vi "GUI_DG535_v2.0.0.vi"() -> ()   [LabVIEW 2020]
uses:
  Device Drivers/DG535/SubVis/mode_typDef.ctl
  Device Drivers/DG535/SubVis/load_typdef.ctl
  DelayControl_For Multiple Channels_535.ctl
  Device Drivers/DG535/SubVis/channels_TypDef_DG535.ctl
  GUI_DG645/DelayControl2.ctl
  Device Drivers/DG645/subVIs/polarity_TypDEf.ctl
  Shared/GUI_Template/GUI_master/tcp_new_data_event.ctl
  Shared/GUI_Template/GUI_master/tcp new data cluster.ctl
panel:
  out "tcp data event":T1
  in  "GUIdevice 1":string="P2-AndorCam"
  in  "stop":bool
  out "UDP error message":string caption="Device Errors"
  in  "Tab Control":T2(tab)
  in  "mode.Channel_C::1":T3
  in  "load.Channel_C::1":T4=enum."50 Ohm" caption="Impedance"
  in  "Delay.Channel_C":T5={"Channel"="C", "reference"=enum."T0", "delay"=0.01} {"delay" format="%+.12f"}
  in  "amplitude.Channel_C::1":dbl=4.0 caption="Amplitude (V)" min=-3.0 max=4.0
  in  "polarity.Channel_C::1":T8=enum."Positive" caption="Polarity"
  in  "mode.Channel_A::1":T3
  in  "load.Channel_A::1":T4=enum."50 Ohm" caption="Impedance"
  in  "Delay.Channel_A":T5={"Channel"="A", "reference"=enum."T0", "delay"=0.002} {"delay" format="%+.12f"}
  in  "amplitude.Channel_A::1":dbl=4.0 caption="Amplitude (V)" min=-3.0 max=4.0
  in  "polarity.Channel_A::1":T8=enum."Positive" caption="Polarity"
  in  "mode.Channel_B::1":T3
  in  "load.Channel_B::1":T4=enum."50 Ohm" caption="Impedance"
  in  "Delay.Channel_B":T5={"Channel"="B", "reference"=enum."T0", "delay"=0.001} {"delay" format="%+.12f"}
  in  "amplitude.Channel_B::1":dbl=4.0 caption="Amplitude (V)" min=-3.0 max=4.0
  in  "polarity.Channel_B::1":T8=enum."Positive" caption="Polarity"
  in  "mode.Channel_D::1":T3
  in  "load.Channel_D::1":T4=enum."50 Ohm" caption="Impedance"
  in  "Delay.Channel_D":T5={"Channel"="D", "reference"=enum."T0", "delay"=0.001} {"delay" format="%+.12f"}
  in  "amplitude.Channel_D::1":dbl=4.0 caption="Amplitude (V)" min=-3.0 max=4.0
  in  "polarity.Channel_D::1":T8=enum."Positive" caption="Polarity"
  in  "mode.Channel_t0::1":T3
  in  "load.Channel_t0::1":T4=enum."50 Ohm" caption="Impedance"
  in  "polarity.Channel_t0::1":T8=enum."Positive" caption="Polarity"
  in  "amplitude.Channel_t0::1":dbl=4.0 caption="Amplitude (V)" min=-3.0 max=4.0
  in  "Delay.Channel_t0":T5={"Channel"="T0", "reference"=enum."T0", "delay"=0.0} {"delay" format="%+.12f"}
  in  "mode.Channel_CD::1":T3
  in  "load.Channel_CD::1":T4=enum."50 Ohm" caption="Impedance"
  in  "amplitude.Channel_CD::1":dbl=4.0 caption="Amplitude (V)" min=-3.0 max=4.0
  in  "amplitude.Channel_AB::1":dbl=4.0 caption="Amplitude (V)" min=-3.0 max=4.0
  in  "load.Channel_AB::1":T4=enum."50 Ohm" caption="Impedance"
  in  "mode.Channel_AB::1":T3
  in  "Refresh Button":bool
  in  "LocalSavingPath::1":path caption="Local Saving Path"
  in  "save::1":bool caption="Save"
  in  "trigger.TrigSource::1":T9(ring) caption="Trigger Source"
  in  "trigger.InternalTrigRate::1":dbl caption="Internal Trigger Rate" min=0.001 max=10000.0
  in  "trigger.BurstPeriod::1":i32 caption="Trigger Burst Period" min=1 max=10
  in  "trigger.TrigSlope::1":enum16{"-ve edge", "+ve edge"}(ring) caption="Slope"
  in  "trigger.BurstCount::1":i32 caption="Trigger Burst Count" min=0 max=10
  in  "trigger.ExternalTrigLevel::1":dbl caption="Exterrnal Trigger Level" min=0.0 max=4.0
  in  "trigger.InputImpedance::1":enum16{"High Z", "50 Ohm"}(ring) caption="Input Impedance"
  in  "Load Local::1":T10(ring) caption="Load Local"
  in  "Save Local::1":T10(ring) caption="Save Local"
  in  "load file::1":bool caption="Load File"
  in  "save::1":bool caption="Save"
  in  "error in":errorcluster
  # "A"
  # "AB"
  # "CD"
  # "C"
  # "="
  # "="
  # "B"
  # "="
  # "D"
  # "="
  # "T0"
  # "="
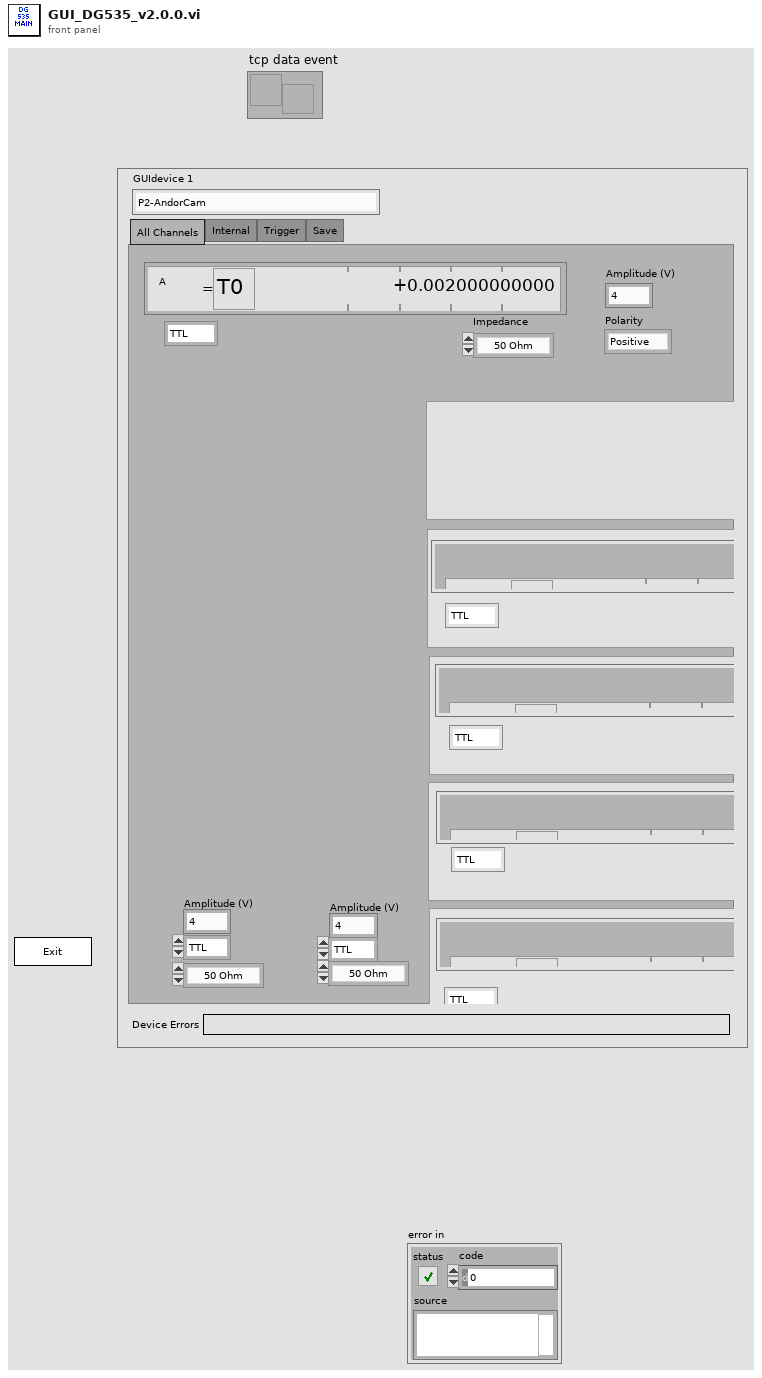
[diagram p1: front panel]
types:
  T1 = typedef "tcp_new_data_event.ctl" = refnum<user-event>
  T2 = enum32{"All Channels", "Internal", "Trigger", "Save"}
  T3 = typedef "mode_typDef.ctl" = enum16{"TTL", "NIM", "ECL", "VAR"}
  T4 = typedef "load_typdef.ctl" = enum16{"High Z", "50 Ohm"}
  T5 = typedef "DelayControl_For Multiple Channels_535.ctl" = cluster{"Channel":string, "reference":T6, "delay":T7}
  T6 = typedef "channels_TypDef_DG535.ctl" = enum16{"T0", "A", "B", "C", "D"}
  T7 = typedef "DelayControl2.ctl" = dbl
  T8 = typedef "polarity_TypDEf.ctl" = enum16{"Negative", "Positive"}
  T9 = enum16{"Internal", "External", "Single Shot", "Burst", "Line"}
  T10 = enum16{"off", "1", "2", "3", "4", "5", "6", "7", "8", "9"}
  T11 = enum32{"invalid app kind", "Development System", "Run Time System", "Student Edition", "Embedded LabVIEW", "Evaluation", "Custom"}
  T12 = typedef "tcp new data cluster.ctl" = cluster{"EventEnum":enum16{"new data", "connection status update"}, "Device name":string}
  T13 = enum32{"Invalid", "Standard", "Closed", "Hidden", "Minimized", "Maximized"}
  T14 = cluster{"Core":cluster{"Current VI Reference":refnum<vi>, "Close Panel on Exit?":bool}, "Your Boolean data":bool, "Your string data":string, "SuperGUI":cluster{"STOP queue":refnum<queue>, "SuperGUI ref":refnum<vi>}}
  T15 = cluster{"STOP queue":refnum<queue>, "SuperGUI ref":refnum<vi>}
  T16 = cluster{"Current VI Reference":refnum<vi>, "Close Panel on Exit?":bool}
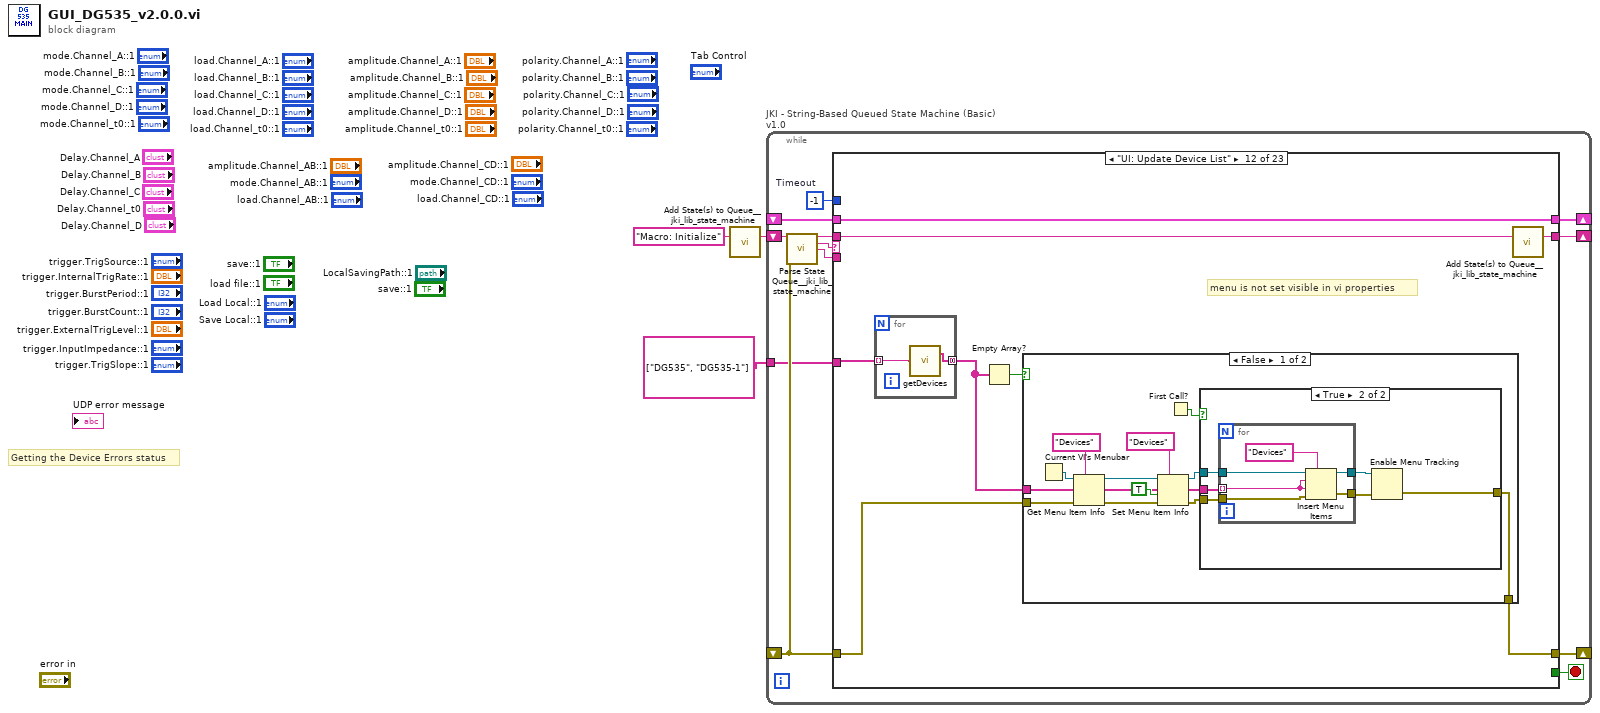
[diagram p0: block diagram]
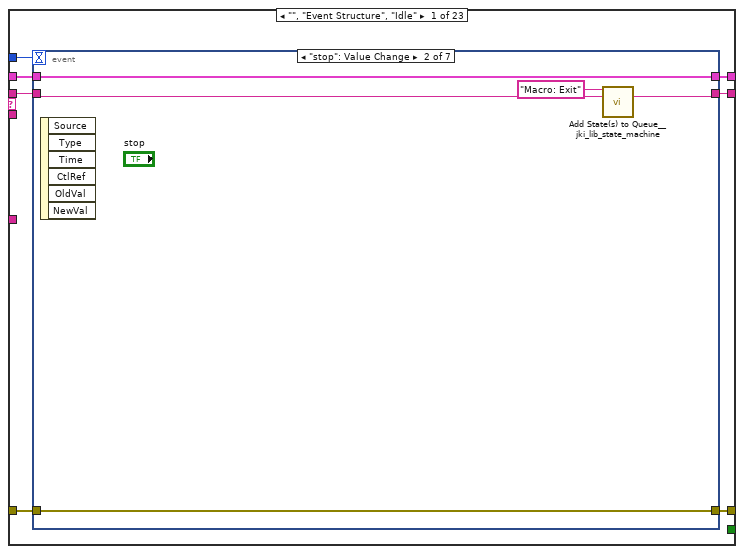
[diagram p2: hidden frame]
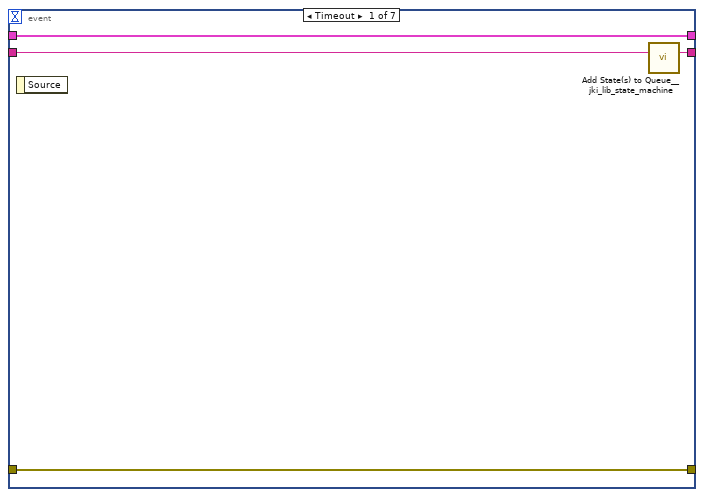
[diagram p3: hidden frame]
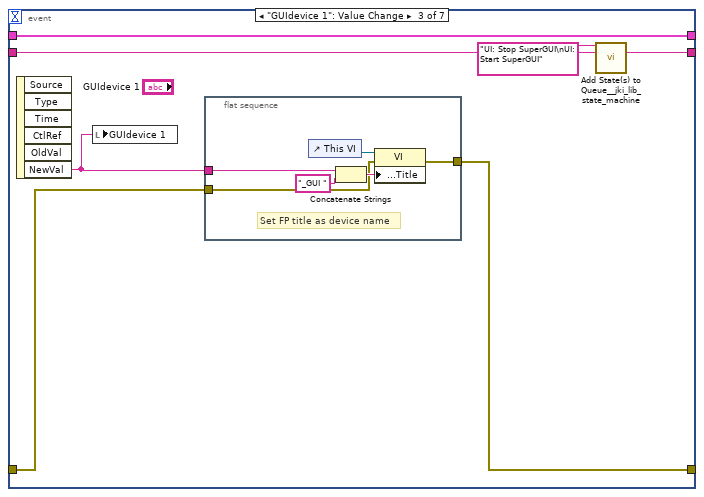
[diagram p4: hidden frame]
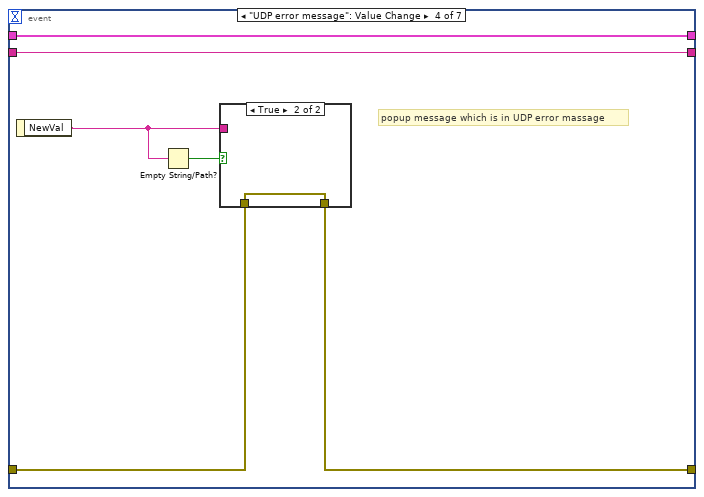
[diagram p5: hidden frame]
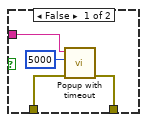
[diagram p6: hidden frame]
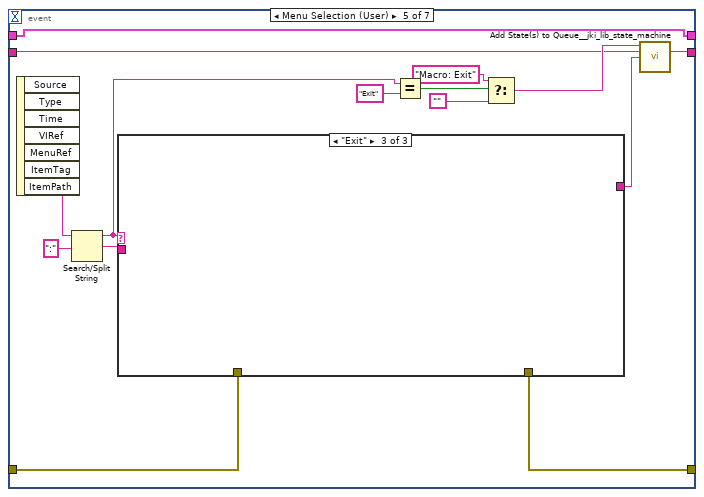
[diagram p7: hidden frame]
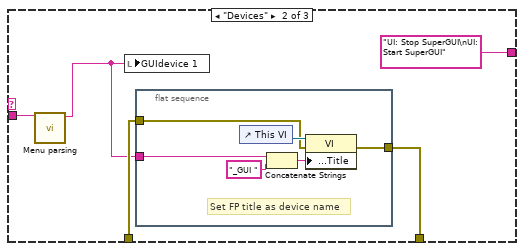
[diagram p9: hidden frame]
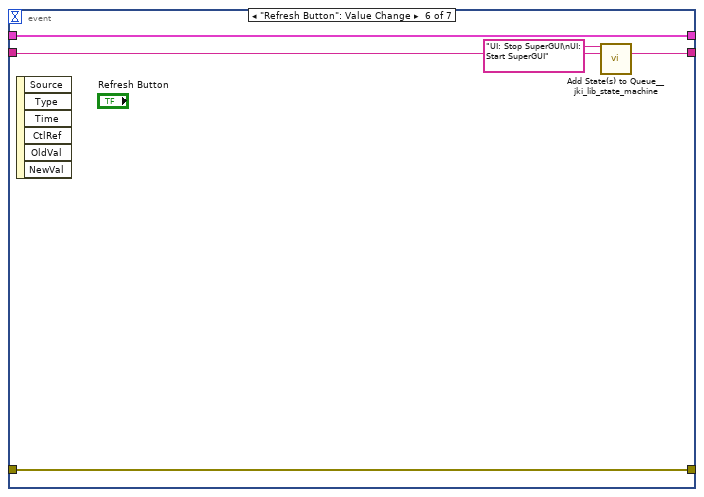
[diagram p10: hidden frame]
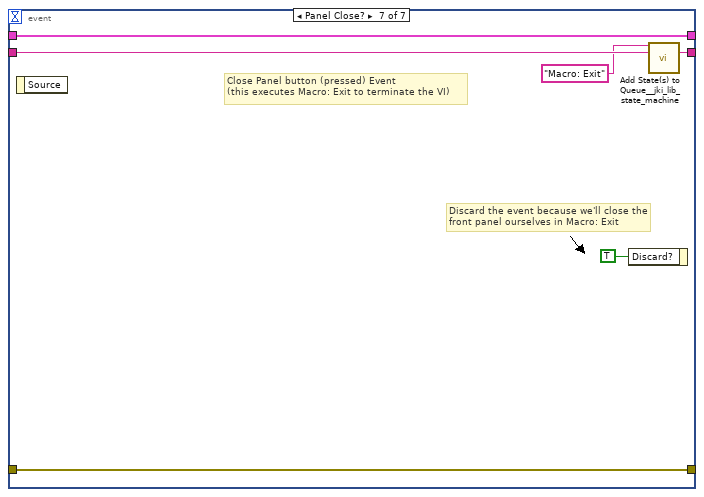
[diagram p11: hidden frame]
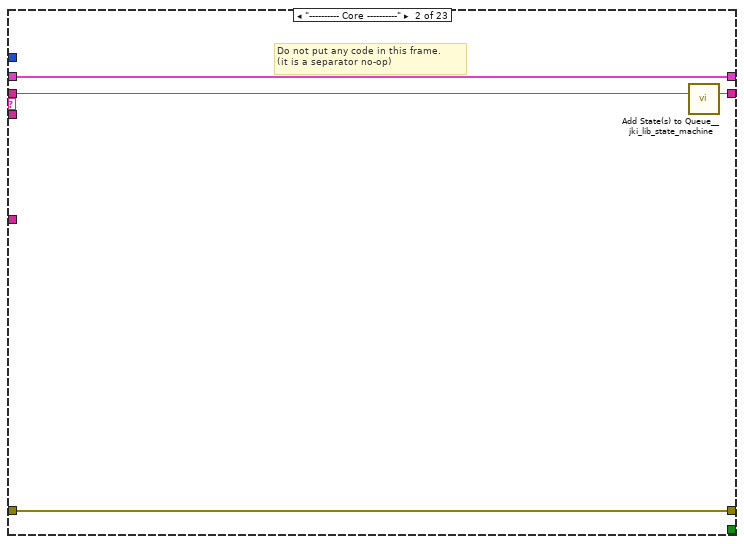
[diagram p12: hidden frame]
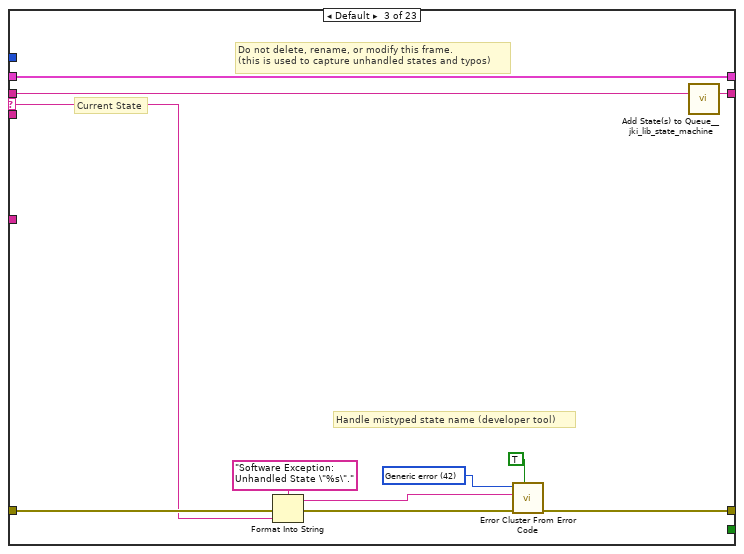
[diagram p13: hidden frame]
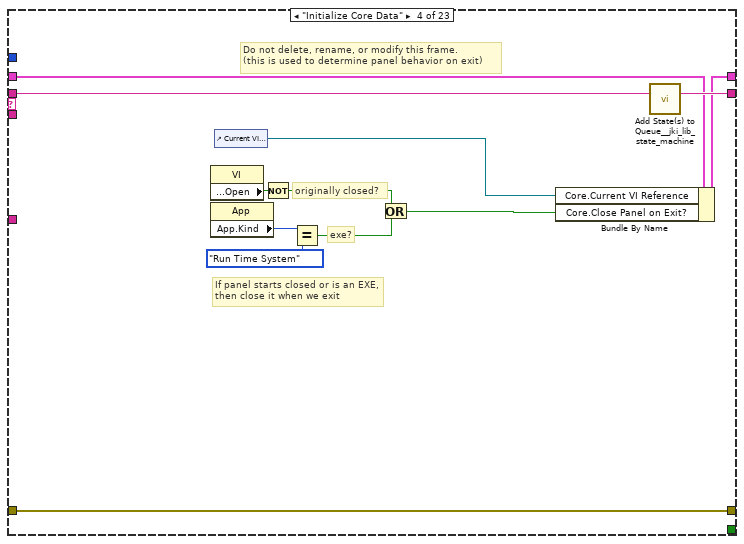
[diagram p14: hidden frame]
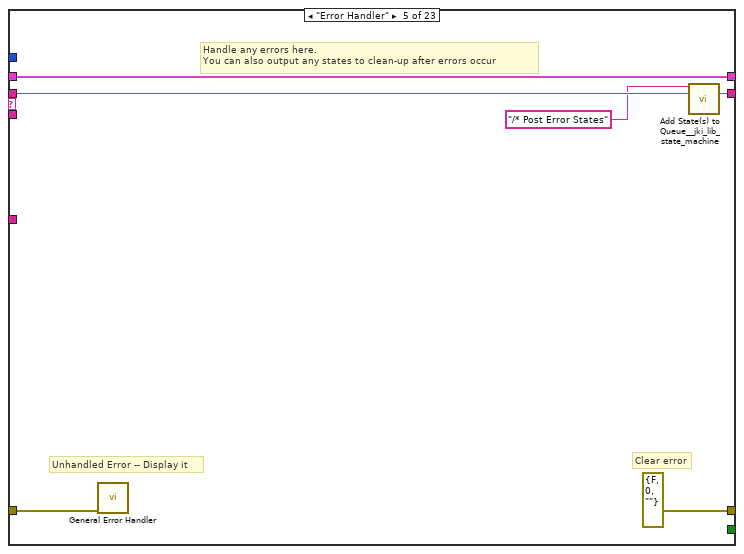
[diagram p15: hidden frame]
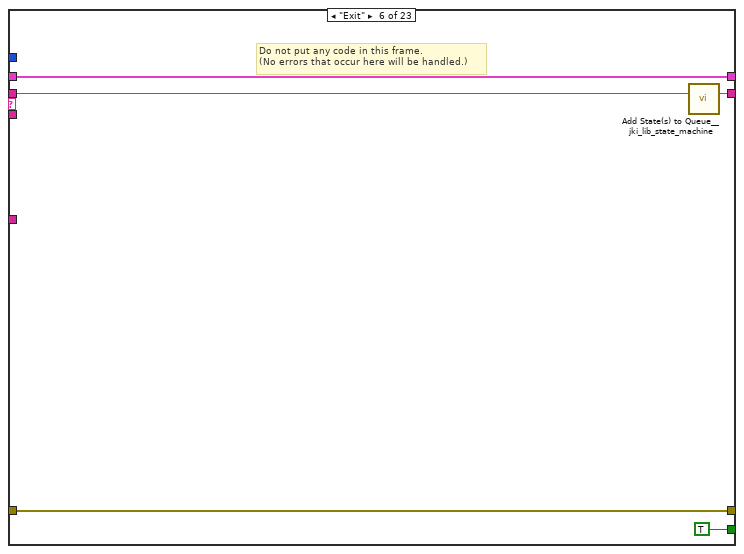
[diagram p16: hidden frame]
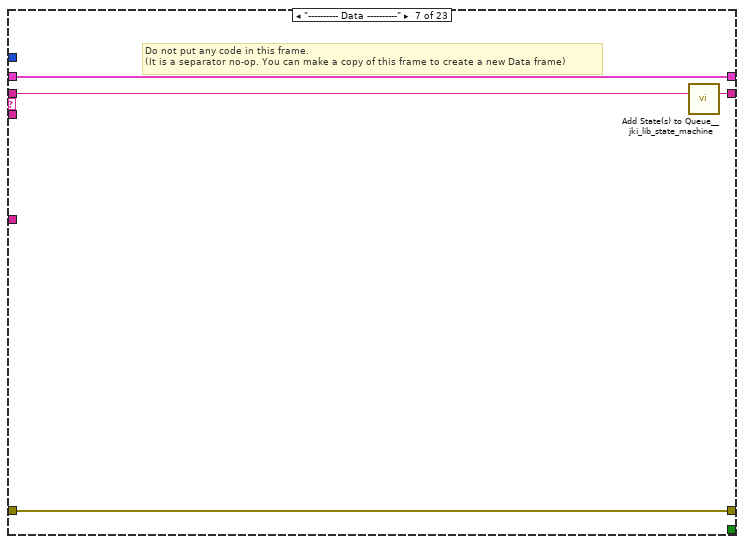
[diagram p17: hidden frame]
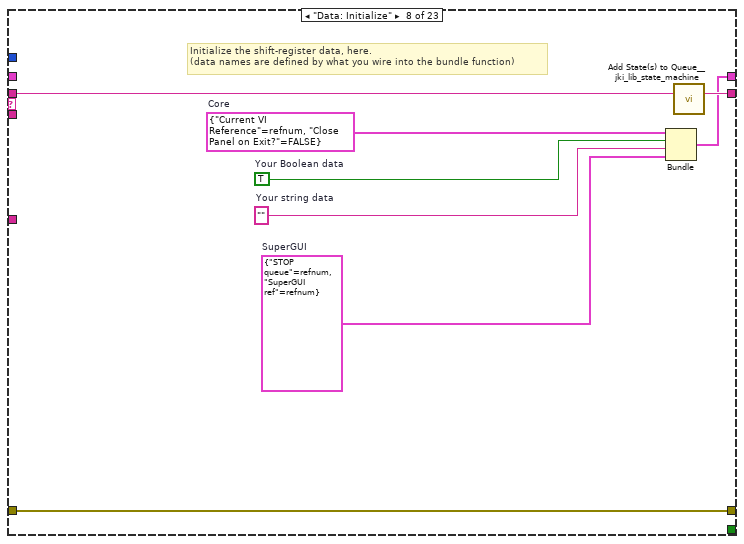
[diagram p18: hidden frame]
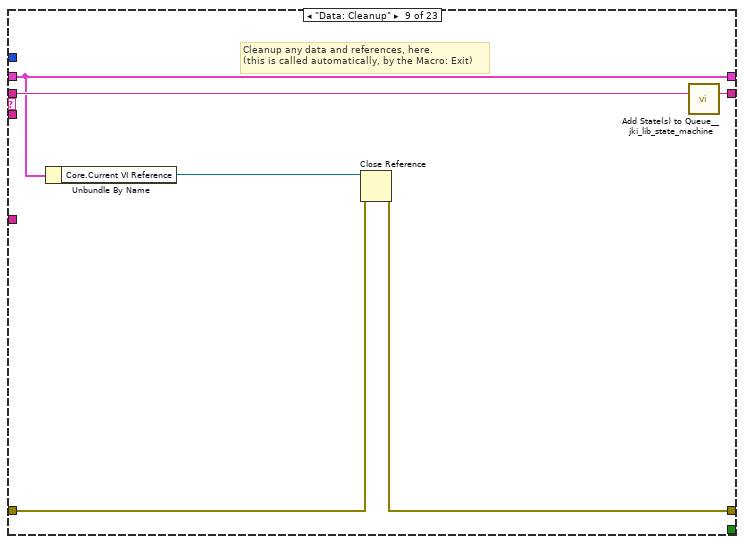
[diagram p19: hidden frame]
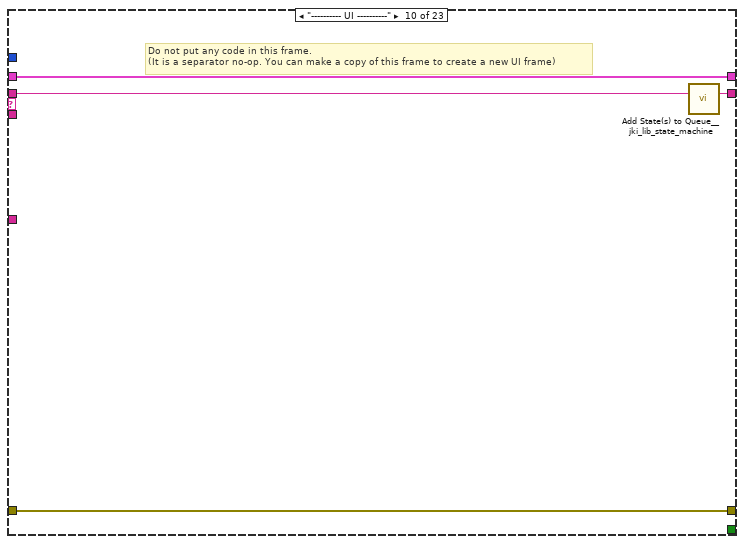
[diagram p20: hidden frame]
diagram:
  # "Getting the Device Errors status"
  n1 = call <vilib>:"Add State(s) to Queue__jki_lib_state_machine.vi"("State(s) in (\"\")"="Macro: Initialize") -> ("States Out"=w3:string)  [unwired: 14 in]
  n2 = while "JKI - String-Based Queued State Machine (Basic) v1.0" {
    shift-right: [w8] -> _
    shift-left: _ -> [w7]
    shift-right: [w11] -> _
    shift-left: _ -> [w5]
    shift-right: [w10] -> _
    shift-left: w3 -> [w12]
    tunnel: string[] ["DG535", "DG535-1"] -> [w4]
    stop <- w9 stop-if-true
    w6 = -1  # Timeout
    n3 = call <vilib>:"Parse State Queue__jki_lib_state_machine.vi"("State Queue"=w12, "Error In (no error)"=w5) -> ("Remaining States"=w14:string, "Current State"=w15:string, "Arguments"=w13:string)  [unwired: 11 in]
    n4 = case shown="\"UI: Update Device List\"" w15 {
      selector: w15 -> [_ _ w99 _ _ _ _ _ _ _ _ _ _ _ _ _ _ _ _ _ _ _ _]
      tunnel: w14 -> [w22 w98 w103 w121 w127 w132 w136 w144 w150 w154 w159 w167 w201 w235 w243 w249 w260 w286 w291 w301 w305 w309 w313]
      tunnel: w13 -> [_ _ _ _ _ _ _ _ _ _ _ _ _ _ _ w244 w254 _ _ _ _ _ _]
      tunnel: w7 -> [w20 w95 w101 w112 w124 w130 w133 _ w145 w151 w157 w165 w199 w226 w238 w247 w256 w283 w288 w298 w302 w306 w310]
      tunnel: [w19 w96 w105 w118 errorcluster {"status"=FALSE, "code"=0, "source"=""} ("error out") w129 w134 w141 w146 w152 w155 w163 w196 w219 w236 w245 w257 w284 w289 w299 w303 w307 w311] -> w11
      tunnel: w5 -> [w18 w96 w104 w118 w123 w129 w134 w141 w147 w152 w156 w164 w197 w220 w237 w246 w258 w284 w289 w299 w303 w307 w311]
      tunnel: [w21 w97 w102 w120 w126 w131 w135 w143 w149 w153 w158 w166 w200 w234 w242 w248 w259 w285 w290 w300 w304 w308 w312] -> w10
      tunnel: [_ _ _ _ _ TRUE _ _ _ _ _ _ _ _ _ _ _ _ _ _ _ _ _] -> w9
      tunnel: [w17 w95 w101 w119 w124 w130 w133 w142 w145 w151 w157 w165 w199 w225 w238 w247 w256 w283 w288 w298 w302 w306 w310] -> w8
      tunnel: w6 -> [w16 _ _ _ _ _ _ _ _ _ _ _ _ _ _ _ _ _ _ _ _ _ _]
      tunnel: w4 -> [_ _ _ _ _ _ _ _ _ _ _ w160 _ _ _ _ _ _ _ _ _ _ _]
      frame "", "Event Structure", "Idle" {
        n5 = event shown="[1] \"stop\": Value Change" {
          selector: _ -> [_ _ _ _ _ _ _]
          dyn-events: _ -> [_ _ _ _ _ _ _]
          timeout: w16 -> [_ _ _ _ _ _ _]
          tunnel: w22 -> [w26 w29 w35 w49 w64 w86 w94]
          tunnel: [w25 w28 w34 w49 w63 w85 w93] -> w21
          tunnel: w20 -> [w23 w31 w38 w50 w70 w88 w91]
          tunnel: [w24 w30 w36 w45 w57 w87 w92] -> w19
          tunnel: w18 -> [w24 w30 w37 w46 w58 w87 w92]
          tunnel: [w23 w31 w38 w50 w70 w88 w91] -> w17
          event Timeout {
            n6 = event-data() -> ()  [unwired: 1 in, 1 out]
            n7 = call <vilib>:"Add State(s) to Queue__jki_lib_state_machine.vi"("State(s) in (\"\")"=w26) -> ("States Out"=w25:string)  [unwired: 14 in]
          }
          event "stop": Value Change {
            n8 = event-data() -> ()  [unwired: 1 in, 6 out]
            n9 = call <vilib>:"Add State(s) to Queue__jki_lib_state_machine.vi"("State(s) in Front (\"\")"="Macro: Exit", "State(s) in (\"\")"=w29) -> ("States Out"=w28:string)  [unwired: 13 in]
          }
          event "GUIdevice 1": Value Change {
            n10 = event-data() -> ("NewVal"=w32:string)  [unwired: 1 in, 5 out]
            n11 = local write "GUIdevice 1"(w32) -> ()
            n12 = flat-sequence {
              tunnel: [w41] -> w36
              tunnel: w37 -> [w40]
              tunnel: w32 -> [w39]
              frame #0 {
                # "Set FP title as device name"
                n13 = control-ref of="This VI"() -> (w44:refnum<vi>)
                n14 = Concatenate Strings(w39, "_GUI ") -> (w43:string)
                n15 = property class="VI"(reference=w44, error in=w40, "Front Panel.Title"=w43) -> (error out=w41:errorcluster)  [unwired: 1 out]
              }
            }
            n16 = call <vilib>:"Add State(s) to Queue__jki_lib_state_machine.vi"("State(s) in Front (\"\")"="UI: Stop SuperGUI\nUI: Start SuperGUI", "State(s) in (\"\")"=w35) -> ("States Out"=w34:string)  [unwired: 13 in]
          }
          event "UDP error message": Value Change {
            # "popup message which is in UDP error massage"
            n17 = event-data() -> ("NewVal"=w47:string)  [unwired: 1 in]
            n18 = Empty String/Path?(string/path=w47) -> (empty?=w48:bool)
            n19 = case shown="True" w48 {
              tunnel: w47 -> [w54 _]
              tunnel: w46 -> [w53 w55]
              tunnel: [w52 w55] -> w45
              frame False {
                n20 = call "Popup with timeout.vi"("error"=w53, "timeout"=u32 5000, "message"=w54) -> ("error out"=w52:errorcluster)  [unwired: 8 in]
              }
              frame True {
              }
            }
          }
          event Menu Selection (User) {
            n21 = event-data() -> ("ItemPath"=w60:string)  [unwired: 1 in, 6 out]
            n22 = Search/Split String(string=w60, search string/char (-)=":") -> (substring before match=w56:string, match + rest of string=w59:string)  [unwired: 1 in, 1 out]
            n23 = case shown="\"Exit\"" w56 {
              tunnel: w59 -> [_ w76 _]
              tunnel: w58 -> [w71 w75 w83]
              tunnel: [w71 w74 w83] -> w57
              tunnel: [_ "UI: Stop SuperGUI\nUI: Start SuperGUI" _] -> w62
              frame "", Default {
              }
              frame "Devices" {
                n24 = call "Menu parsing.vi"("ItemPath 3"=w76) -> ("ItemPath 2"=w72:string)  [unwired: 9 in, 1 out]
                n25 = local write "GUIdevice 1"(w72) -> ()
                n26 = flat-sequence {
                  tunnel: [w79] -> w74
                  tunnel: w75 -> [w78]
                  tunnel: w72 -> [w77]
                  frame #0 {
                    # "Set FP title as device name"
                    n27 = control-ref of="This VI"() -> (w82:refnum<vi>)
                    n28 = Concatenate Strings(w77, "_GUI ") -> (w81:string)
                    n29 = property class="VI"(reference=w82, error in=w78, "Front Panel.Title"=w81) -> (error out=w79:errorcluster)  [unwired: 1 out]
                  }
                }
              }
              frame "Exit" {
              }
            }
            n30 = Equal?(x=w56, y="Exit") -> (x = y?=w68:bool)
            n31 = Select(t="Macro: Exit", s=w68, f="") -> (s? t:f=w65:string)
            n32 = call <vilib>:"Add State(s) to Queue__jki_lib_state_machine.vi"("State(s) in Front (\"\")"=w65, "State(s) in (\"\")"=w64, "State(s) at Back (\"\")"=w62) -> ("States Out"=w63:string)  [unwired: 12 in]
          }
          event "Refresh Button": Value Change {
            n33 = event-data() -> ()  [unwired: 1 in, 6 out]
            n34 = call <vilib>:"Add State(s) to Queue__jki_lib_state_machine.vi"("State(s) in Front (\"\")"="UI: Stop SuperGUI\nUI: Start SuperGUI", "State(s) in (\"\")"=w86) -> ("States Out"=w85:string)  [unwired: 13 in]
          }
          event Panel Close? {
            # "Discard the event because we'll close the front panel ourselves in Macro: Exit"
            # "Close Panel button (pressed) Event\n(this executes Macro: Exit to terminate the VI)"
            n35 = event-data() -> ()  [unwired: 1 in, 1 out]
            n36 = event-data("Discard?"=TRUE) -> ()  [unwired: 1 in, 1 out]
            n37 = call <vilib>:"Add State(s) to Queue__jki_lib_state_machine.vi"("State(s) in Front (\"\")"="Macro: Exit", "State(s) in (\"\")"=w94) -> ("States Out"=w93:string)  [unwired: 13 in]
          }
        }
      }
      frame "---------- Core ----------" {
        # "Do not put any code in this frame.\n(it is a separator no-op)"
        n38 = call <vilib>:"Add State(s) to Queue__jki_lib_state_machine.vi"("State(s) in (\"\")"=w98) -> ("States Out"=w97:string)  [unwired: 14 in]
      }
      frame Default {
        w108 = 42 items=["No error", "Argument error", "Memory is full", "Out of zone", "End of file", "File already open", "Generic file I/O error", "File not found", "File permission error", "Disk is full", "Duplicate path", "Too many files open", "System feature not enabled", "Resource file not found", "Cannot add resource", "Resource not found", "Image not found", "Image memory error", "Pen does not exist", "Config type invalid", "Config token not found", "Config parse error", "Config memory error", "Bad external code format", "Bad external code offset", "External code not present", "Null window", "Destroy window error", "Null menu", "Print aborted", "Bad print record", "Print driver error", "Windows error during printing", "Memory error during printing", "Print dialog error", "Generic print error", "Invalid device refnum", "Device not found", "Device parameter error", "Device unit error", "Cannot open device", "Device call aborted", "Generic error", "Cancelled by user", "Object ID too low", "Object ID too high", "Object not in heap", "Unknown heap", "Unknown object (invalid DefProc)", "Unknown object (DefProc not in table)", "Message out of range", "Invalid (null) method", "Unknown message", "Manager call not supported", "Bad address", "Network operation in progress", "Network operation timed out", "Connection is busy", "Network attribute not supported", "Network error", "Address in use", "System out of memory", "Connection aborted", "Connection refused", "Not connected", "Already connected", "Connection closed", "Initialization error (interapplication manager)", "Bad occurrence", "Wait on unbound occurrence handler", "Occurrence queue overflow", "Datalog type conflict", "Unused", "Unrecognized type (interapplication manager)", "Memory corrupt", "Failed to make temporary DLL", "Old CIN version", "Drag socket not found", "Failed to load drop-object", "Failed to register OLE object", "Failed to release OLE object", "Format specifier type mismatch", "Unknown format specifier", "Too few format specifiers", "Too many format specifiers", "Scan failed", "Newer CIN version", "Error converting to variant", "Runtime menu error", "Password tampered", "Variant attribute not found", "Incompatible variant data type", "Event data is not available", "Event Store is not present", "Occurrence is not found", "Event Queue is not created", "Event info is not available", "Refnum passed is NULL", "Error retrieving Class GUID", "Error retrieving CoClass GUID", "Error retrieving TypeLib GUID.", "Bad built application magic bytes.", "Specific driver is different from the specific driver associated with the Logical Name.", "There is no session opened to the class driver.", "Max Error", "MAX - Error with config objects", "MAX - Error loading configuration", "MAX - Group not supported"]
        # "Current State"
        # "Do not delete, rename, or modify this frame.\n(this is used to capture unhandled states and typos)"
        # "Handle mistyped state name (developer tool)"
        n39 = Format Into String(format string="Software Exception: Unhandled State \"%s\"." ("message"), error in=w104, w99) -> (resulting string=w107:string, error out=w106:errorcluster)  [unwired: 1 in]
        n40 = call <vilib>:"Error Cluster From Error Code.vi"("show call chain? (False)"=TRUE, "error in (no error)"=w106, "error message (\"\")"=w107, "error code (0)"=w108) -> ("error out"=w105:errorcluster)  [unwired: 5 in]
        n41 = call <vilib>:"Add State(s) to Queue__jki_lib_state_machine.vi"("State(s) in (\"\")"=w103) -> ("States Out"=w102:string)  [unwired: 14 in]
      }
      frame "Initialize Core Data" {
        # "Do not delete, rename, or modify this frame.\n(this is used to determine panel behavior on exit)"
        # "originally closed?"
        # "exe?"
        # "If panel starts closed or is an EXE, then close it when we exit"
        n42 = property class="VI"() -> ("Front Panel.Open"=w117:bool)  [unwired: 2 in, 2 out]
        n43 = property class="App"() -> ("App.Kind"=w116:T11)  [unwired: 2 in, 2 out]
        n44 = control-ref of="Current VI Reference"() -> (w110:refnum<vi>)
        n45 = Not(x=w117) -> (.not. x?=w114:bool)
        n46 = Equal?(x=w116, y=T11."Run Time System" ("Application:Kind")) -> (x = y?=w113:bool)
        n47 = Or(x=w114, y=w113) -> (x .or. y?=w111:bool)
        n48 = Bundle By Name(cluster=w112, "Core.Current VI Reference"=w110, "Core.Close Panel on Exit?"=w111) -> (w119:T14)
        n49 = call <vilib>:"Add State(s) to Queue__jki_lib_state_machine.vi"("State(s) in (\"\")"=w121) -> ("States Out"=w120:string)  [unwired: 14 in]
      }
      frame "Error Handler" {
        # "Unhandled Error -- Display it"
        # "Handle any errors here.\nYou can also output any states to clean-up after errors occur"
        # "Clear error"
        n50 = call <vilib>:"General Error Handler.vi"("error in (no error)"=w123) -> ()  [unwired: 10 in, 5 out]
        n51 = call <vilib>:"Add State(s) to Queue__jki_lib_state_machine.vi"("State(s) in Front (\"\")"="/* Post Error States", "State(s) in (\"\")"=w127) -> ("States Out"=w126:string)  [unwired: 13 in]
      }
      frame "Exit" {
        # "Do not put any code in this frame.\n(No errors that occur here will be handled.)"
        n52 = call <vilib>:"Add State(s) to Queue__jki_lib_state_machine.vi"("State(s) in (\"\")"=w132) -> ("States Out"=w131:string)  [unwired: 14 in]
      }
      frame "---------- Data ----------" {
        # "Do not put any code in this frame.\n(It is a separator no-op. You can make a copy of this frame to create a new Data frame)"
        n53 = call <vilib>:"Add State(s) to Queue__jki_lib_state_machine.vi"("State(s) in (\"\")"=w136) -> ("States Out"=w135:string)  [unwired: 14 in]
      }
      frame "Data: Initialize" {
        w137 = T15 {"STOP queue"=refnum, "SuperGUI ref"=refnum}  # SuperGUI
        w138 = T16 {"Current VI Reference"=refnum, "Close Panel on Exit?"=FALSE}  # Core
        w140 = TRUE  # Your Boolean data
        w139 = ""  # Your string data
        # "Initialize the shift-register data, here.\n(data names are defined by what you wire into the bundle function)"
        n54 = Bundle("Core"=w138, "Your Boolean data"=w140, "Your string data"=w139, "SuperGUI"=w137) -> (w142:T14)  [unwired: 1 in]
        n55 = call <vilib>:"Add State(s) to Queue__jki_lib_state_machine.vi"("State(s) in (\"\")"=w144) -> ("States Out"=w143:string)  [unwired: 14 in]
      }
      frame "Data: Cleanup" {
        # "Cleanup any data and references, here.\n(this is called automatically, by the Macro: Exit)"
        n56 = Unbundle By Name(w145) -> ("Core.Current VI Reference"=w148:refnum<vi>)
        n57 = Close Reference(reference=w148, error in (no error)=w147) -> (error out=w146:errorcluster)
        n58 = call <vilib>:"Add State(s) to Queue__jki_lib_state_machine.vi"("State(s) in (\"\")"=w150) -> ("States Out"=w149:string)  [unwired: 14 in]
      }
      frame "---------- UI ----------" {
        # "Do not put any code in this frame.\n(It is a separator no-op. You can make a copy of this frame to create a new UI frame)"
        n59 = call <vilib>:"Add State(s) to Queue__jki_lib_state_machine.vi"("State(s) in (\"\")"=w154) -> ("States Out"=w153:string)  [unwired: 14 in]
      }
      frame "UI: Initialize" {
        # "Initialize the User Interface, here.\n(this is called automatically, by the Macro: Init)"
        n60 = call <userlib>:"Fit VI window to Largest Dec__ogtk.vi"("error in (no error)"=w156) -> ("error out"=w155:errorcluster)  [unwired: 5 in, 1 out]
        n61 = call <vilib>:"Add State(s) to Queue__jki_lib_state_machine.vi"("State(s) in (\"\")"=w159) -> ("States Out"=w158:string)  [unwired: 14 in]
      }
      frame "UI: Update Device List" {
        # "menu is not set visible in vi properties"
        n62 = for {
          tunnel: [w168] -> w161 mode=concatenating
          tunnel: w160 -> [w169] mode=indexing
          n63 = call "getDevices.vi"("Device Class"=w169) -> ("All Devices"=w168:string[])  [unwired: 1 out]
        }
        n64 = Empty Array?(array=w161) -> (empty?=w162:bool)
        n65 = case shown="False" w162 {
          tunnel: w164 -> [w172 w195]
          tunnel: [w171 w195] -> w163
          tunnel: w161 -> [w170 _]
          frame False {
            n66 = Current VI's Menubar() -> (w175:refnum<k9>)
            n67 = Get Menu Item Info(7:"Devices" ("item tag"), 8:w172, 11:w175) -> (0:w181:errorcluster, 3:w177:refnum<k9>)  [unwired: 5 out]
            n68 = Set Menu Item Info(7:"Devices" ("item tag"), 8:w181, 9:TRUE ("enabled"), 11:w177) -> (0:w180:errorcluster, 3:w179:refnum<k9>)  [unwired: 3 in]
            n69 = First Call?() -> (First Call?: T/F=w173:bool)
            n70 = case shown="True" w173 {
              tunnel: w179 -> [_ w187]
              tunnel: w170 -> [_ w186]
              tunnel: w180 -> [w182 w184]
              tunnel: [w182 w183] -> w171
              frame False {
              }
              frame True {
                n71 = for {
                  tunnel: [w194] -> w188
                  tunnel: w186 -> [w192] mode=indexing
                  tunnel: w187 -> [w191]
                  tunnel: [w190] -> w185
                  tunnel: w184 -> [w189]
                  n72 = Insert Menu Items(5:"Devices" ("menu tag"), 6:w189, 7:w192, 8:w192, 9:w191) -> (0:w190:errorcluster, 3:w194:refnum<k9>)  [unwired: 1 in, 1 out]
                }
                n73 = Enable Menu Tracking(2:w185, 4:w188) -> (0:w183:errorcluster)  [unwired: 1 in, 1 out]
              }
            }
          }
          frame True {
          }
        }
        n74 = call <vilib>:"Add State(s) to Queue__jki_lib_state_machine.vi"("State(s) in (\"\")"=w167) -> ("States Out"=w166:string)  [unwired: 14 in]
      }
      frame "UI: Get Device Name" {
        n75 = First Call?() -> (First Call?: T/F=w198:bool)
        n76 = case shown="True" w198 {
          tunnel: w197 -> [w202 w204]
          tunnel: [w202 w203] -> w196
          frame False {
          }
          frame True {
            n77 = disable-structure "Get Device name from control for vi mode\nand command line arg for exe" shown="RUN_TIME_ENGINE==True" {
              disable-tunnel: w204 -> [_ w206]
              disable-tunnel: [_ w205] -> w203
              frame condition #0 (active) {
              }
              frame condition #1 {
                n78 = control-ref of="This Application"() -> (w214:refnum<vi>)
                n79 = property class="App"(reference=w214) -> ("App.Args"=w213:string[])  [unwired: 1 in, 2 out]
                n80 = Index Array(array=w213, index #1=1 ("index")) -> (element #1=w207:string)  [unwired: 2 in, 2 out]
                n81 = Empty String/Path?(string/path=w207) -> (empty?=w211:bool)
                n82 = control-ref of="This VI"() -> (w210:refnum<vi>)
                n83 = case shown="False" w211 {
                  tunnel: w207 -> [w215 _]
                  frame False {
                    n84 = local write "GUIdevice 1"(w215) -> ()
                  }
                  frame True {
                  }
                }
                n85 = Concatenate Strings(w207, "_GUI ") -> (w209:string)
                n86 = property class="VI"(reference=w210, error in=w206, "Front Panel.Title"=w209) -> (error out=w205:errorcluster)  [unwired: 1 out]
              }
            }
          }
        }
        n87 = call <vilib>:"Add State(s) to Queue__jki_lib_state_machine.vi"("State(s) in (\"\")"=w201) -> ("States Out"=w200:string)  [unwired: 14 in]
      }
      frame "UI: Start SuperGUI" {
        # "create stop queue for supergui and its clones"
        # "x100 abort will be dependent on caller VI\nx80 abort will be independent of caller vi, this will abort vi when labview is closed."
        # "Start SuperGUI asynchronous way"
        n88 = vi-ref "GUI_Master_subvi_reentrant_queues.vi"() -> (w218:refnum<vi>)
        n89 = property class="VI"(reference=w218) -> ("Path"=w217:path)  [unwired: 1 in, 2 out]
        n90 = Create User Event(user event datatype=T12 {"EventEnum"=enum."new data", "Device name"="Device name"} ("New Event"), error in=w220) -> (user event=w221:refnum<user-event>, error out=w227:errorcluster)
        "tcp data event" <- w221
        n91 = control-ref of="This Application"() -> (w224:refnum<vi>)
        n92 = control-ref of="This VI"() -> (w223:refnum<vi>)
        n93 = Open VI Reference(type specifier VI Refnum (for type only)=refnum<vi> refnum, vi path=w217, options=256) -> (vi reference=w233:refnum<vi>, error out=w232:errorcluster)  [unwired: 3 in]
        n94 = register-events(w221) -> ()  [unwired: 2 in, 2 out]
        n95 = call "supergui create stop queue.vi"() -> ("STOP Queue out"=w229:refnum<queue>)  [unwired: 11 in]
        n96 = Current VI's Menubar() -> (w222:refnum<k9>)
        n97 = call-by-ref "Start Asynchronous Call"(reference=w233, error in=w232, "STOP Queue in"=w229, "This Application"=w224, 8:"error in (no error)"=w227, "tcp data event"=w221, "Caller menu reference"=w222, "Caller VI ref"=w223) -> (reference out=w216:refnum<vi>, error out=w219:errorcluster)  [unwired: 5 in, 1 out]
        n98 = Bundle By Name(cluster=w226, "SuperGUI.SuperGUI ref"=w216, "SuperGUI.STOP queue"=w229) -> (w225:T14)
        n99 = call <vilib>:"Add State(s) to Queue__jki_lib_state_machine.vi"("State(s) in (\"\")"=w235) -> ("States Out"=w234:string)  [unwired: 14 in]
      }
      frame "UI: Stop SuperGUI" {
        # "Stop Supergui Clone and wait until it exit properly"
        n100 = Unbundle By Name(w238) -> ("SuperGUI.SuperGUI ref"=w240:refnum<vi>, "SuperGUI.STOP queue"=w239:refnum<queue>)
        n101 = Release Queue(queue=w239, error in (no error)=w237) -> (error out=w241:errorcluster)  [unwired: 1 in, 2 out]
        n102 = call-by-ref "Wait On Asynchronous Call"(reference=w240, error in=w241) -> ("error out"=w236:errorcluster)  [unwired: 11 in, 2 out]
        n103 = call <vilib>:"Add State(s) to Queue__jki_lib_state_machine.vi"("State(s) in (\"\")"=w243) -> ("States Out"=w242:string)  [unwired: 14 in]
      }
      frame "UI: Cursor Set" {
        # "Argument"
        # "Set and Unset Cursor Busy.\n(Usage: \"UI: Cursor Set >> Busy|Idle\")"
        n104 = case shown="\"Idle\", Default" w244 {
          tunnel: w246 -> [w251 w253]
          tunnel: [w250 w252] -> w245
          frame "Idle", Default {
            n105 = call <vilib>:"Unset Busy.vi"("error in (no error)"=w251) -> ("error out"=w250:errorcluster)  [unwired: 10 in]
          }
          frame "Busy" {
            n106 = call <vilib>:"Set Busy.vi"("error in (no error)"=w253) -> ("error out"=w252:errorcluster)  [unwired: 9 in, 1 out]
          }
        }
        n107 = call <vilib>:"Add State(s) to Queue__jki_lib_state_machine.vi"("State(s) in (\"\")"=w249) -> ("States Out"=w248:string)  [unwired: 14 in]
      }
      frame "UI: Front Panel State" {
        # "Argument"
        # "Set Front Panel Open or Closed\n(Usage: \"UI: Front Panel State >> Open|Close\")"
        n108 = Unbundle By Name(w256) -> ("Core.Current VI Reference"=w255:refnum<vi>)
        n109 = case shown="\"Close\"" w254 {
          tunnel: w258 -> [w264 w277]
          tunnel: [w266 w278] -> w257
          tunnel: w255 -> [w265 w275]
          frame "Open", Default {
            n110 = property class="VI"(reference=w265, error in=w264) -> (reference out=w262:refnum<vi>, error out=w263:errorcluster, "Front Panel.Open"=w261:bool)
            n111 = case shown="False" w261 {
              tunnel: [w269 w272] -> w266
              tunnel: w263 -> [w268 w272]
              tunnel: w262 -> [w267 _]
              frame False {
                n112 = invoke class="VI" method="FP.Open"(reference=w267, error in=w268, "Activate"=TRUE, "State"=T13."Standard") -> (error out=w269:errorcluster)  [unwired: 1 in, 4 out]
              }
              frame True {
              }
            }
          }
          frame "Close" {
            n113 = property class="VI"(reference=w275, error in=w277) -> (reference out=w274:refnum<vi>, error out=w276:errorcluster, "Front Panel.Open"=w273:bool)
            n114 = case shown="True" w273 {
              tunnel: [w279 w282] -> w278
              tunnel: w276 -> [w279 w281]
              tunnel: w274 -> [_ w280]
              frame False {
              }
              frame True {
                n115 = invoke class="VI" method="FP.Close"(reference=w280, error in=w281) -> (error out=w282:errorcluster)  [unwired: 1 in, 2 out]
              }
            }
          }
        }
        n116 = call <vilib>:"Add State(s) to Queue__jki_lib_state_machine.vi"("State(s) in (\"\")"=w260) -> ("States Out"=w259:string)  [unwired: 14 in]
      }
      frame "---------- Macro ----------" {
        # "Do not put any code in this frame.\n(It is a separator no-op. You can make a copy of this frame to create a new Macro frame)"
        n117 = call <vilib>:"Add State(s) to Queue__jki_lib_state_machine.vi"("State(s) in (\"\")"=w286) -> ("States Out"=w285:string)  [unwired: 14 in]
      }
      frame "Macro: Initialize" {
        # "Initialization Macro\n(This is called once, when the VI starts)"
        n118 = call <vilib>:"Add State(s) to Queue__jki_lib_state_machine.vi"("State(s) in Front (\"\")"="Data: Initialize\nInitialize Core Data\nUI: Initialize\nUI: Update Device List\nUI: Get Device Name\nUI: Start SuperGUI\nUI: Front Panel State >> Open", "State(s) in (\"\")"=w291) -> ("States Out"=w290:string)  [unwired: 13 in]
      }
      frame "Macro: Exit" {
        # "Exit Macro\n(This is called once, when the VI exits)"
        n119 = Unbundle By Name(w298) -> ("Core.Close Panel on Exit?"=w297:bool)
        n120 = Select(t="UI: Front Panel State >> Close", s=w297, f="") -> (s? t:f=w294:string)
        n121 = call <vilib>:"Add State(s) to Queue__jki_lib_state_machine.vi"("State(s) in (\"\")"=w294, "State(s) at Back (\"\")"="Data: Cleanup\nExit") -> ("States Out"=w292:string)  [unwired: 13 in]
        n122 = call <vilib>:"Add State(s) to Queue__jki_lib_state_machine.vi"("State(s) in Front (\"\")"=w292, "State(s) in (\"\")"=w301) -> ("States Out"=w300:string)  [unwired: 13 in]
      }
      frame "---------- New Category ----------" {
        # "Template Separator\n(You can make a copy of, or modify, this frame)"
        n123 = call <vilib>:"Add State(s) to Queue__jki_lib_state_machine.vi"("State(s) in (\"\")"=w305) -> ("States Out"=w304:string)  [unwired: 14 in]
      }
      frame "New Category: 1" {
        # "Your code here.\n(You can make a copy of, or modify, this frame)"
        n124 = call <vilib>:"Add State(s) to Queue__jki_lib_state_machine.vi"("State(s) in (\"\")"=w309) -> ("States Out"=w308:string)  [unwired: 14 in]
      }
      frame "New Category: 2" {
        # "Your code here.\n(You can make a copy of, or modify, this frame)"
        n125 = call <vilib>:"Add State(s) to Queue__jki_lib_state_machine.vi"("State(s) in (\"\")"=w313) -> ("States Out"=w312:string)  [unwired: 14 in]
      }
    }
  }
